vi "Query Auto Load Compensation.vi"(6 "channel":i32=1 min=1 max=4, 8 "error in (no error)":errorcluster, 11 "VISA resource name":refnum<visa-resource-name>) -> (0 "error Out (no error)":errorcluster, 2 "auto load compensation":bool, 3 "VISA resource name out":refnum<visa-resource-name>)   [LabVIEW 2019, in "Pulse Rider PG-1000.lvlib"]
doc: "Query the automatic calculation of the load impedance for the selected output channel. If the load compensation is set to ON, the value set through the command Load Impedence will be ignored.\n\nchannel: the output channel int from 1 to 4"
uses:
  <instrlib>/Pulse Rider PG-1000/Pulse Rider PG-1000.lvlib
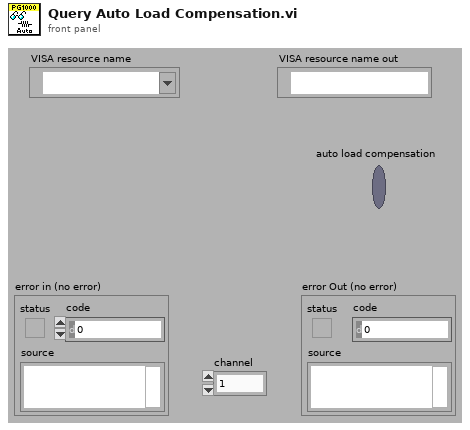
[diagram p1: front panel]
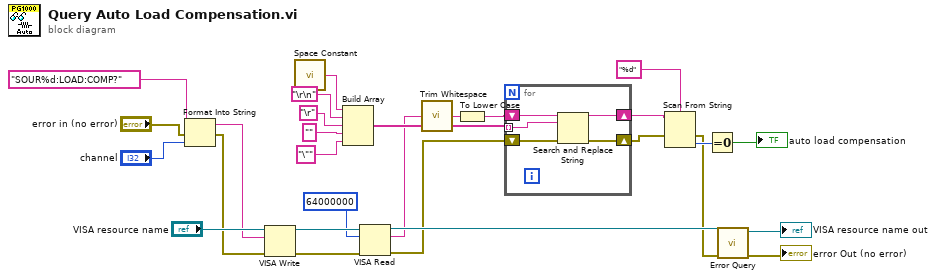
[diagram p0: block diagram]
diagram:
  n1 = Format Into String(format string="SOUR%d:LOAD:COMP?", error in="error in (no error)", "channel") -> (resulting string=w10:string, error out=w4:errorcluster)  [unwired: 1 in]
  n2 = VISA Write(VISA resource name="VISA resource name", write buffer=w10, error in (no error)=w4) -> (VISA resource name out=w25:refnum<visa-resource-name>, error out=w24:errorcluster)  [unwired: 1 out]
  n3 = call <vilib>:"Space Constant.vi"() -> ("String"=w21:string)
  n4 = Build Array(w21, "\r\n", "\r", "", "\"") -> (w16:string[])
  n5 = VISA Read(VISA resource name=w25, byte count=u32 64000000, error in (no error)=w24) -> (VISA resource name out=w22:refnum<visa-resource-name>, read buffer=w14:string, error out=w3:errorcluster)  [unwired: 1 out]
  n6 = call <vilib>:"Trim Whitespace.vi"("string"=w14) -> ("trimmed string"=w15:string)  [unwired: 1 in]
  n7 = To Lower Case(string=w15) -> (all lower case string=w13:string)
  n8 = for {
    tunnel: w16 -> [w31] mode=indexing
    shift-right: [w33] -> w9
    shift-left: w13 -> [w32]
    shift-right: [w29] -> w2
    shift-left: w3 -> [w30]
    n9 = Search and Replace String(input string=w32, search string=w31, error in=w30) -> (result string=w33:string, error out=w29:errorcluster)  [unwired: 5 in, 2 out]
  }
  n10 = Scan From String(format string="%d", input string=w9, error in=w2) -> (error out=w1:errorcluster, output 1=w7:i32)  [unwired: 2 in, 2 out]
  n11 = Equal To 0?(x=w7) -> (x = 0?=→"auto load compensation":bool)
  n12 = call <instrlib>:"Error Query.vi"("error in (no error)"=w1, "VISA resource name"=w22) -> ("error out"=→"error Out (no error)":errorcluster, "VISA resource name out"=→"VISA resource name out":refnum<visa-resource-name>)  [unwired: 6 in, 2 out]
